vi "Calculate Channel Value.vi"(9 "Digital":bool=TRUE, 10 "Remaining Time":dbl, 11 "Step Settings":T1) -> (3 "Values to Write":dbl[](array[numeric]))   [LabVIEW 2020, in "Sequencer with Output Values.lvlib" / "Sequencer with Output Values.lvclass"]
uses:
  Sequencer with Output Values.lvclass
  Step Settings.ctl
  Global Strings.vi
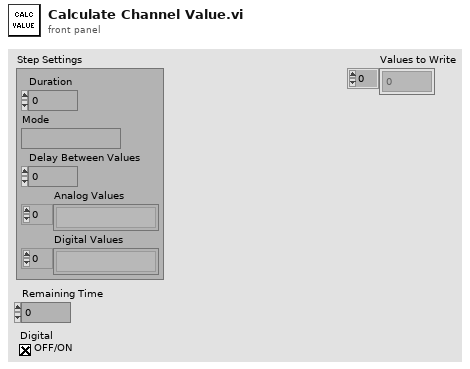
[diagram p1: front panel]
types:
  T1 = typedef "Sequencer with Output Values.lvlib/Sequencer with Output Values.lvclass/Step Settings.ctl" = cluster{"Duration":dbl, "Mode":string, "Delay Between Values":dbl, "Analog Values":string[], "Digital Values":string[]}
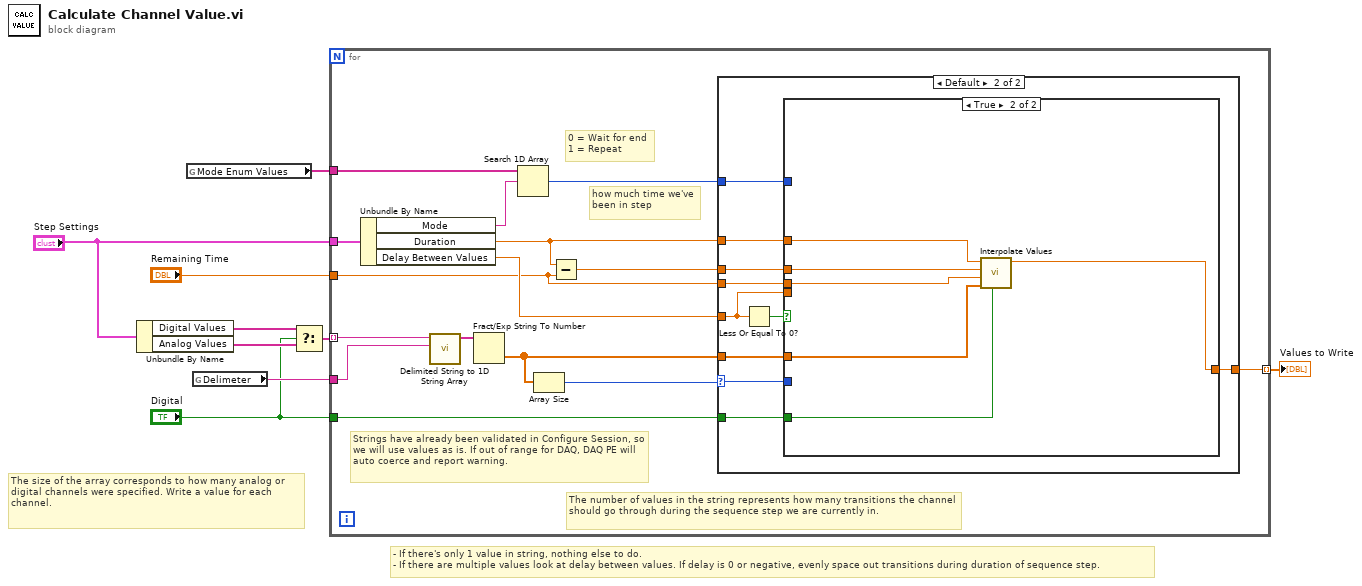
[diagram p0: block diagram]
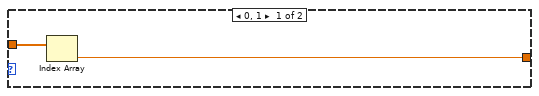
[diagram p2: hidden frame]
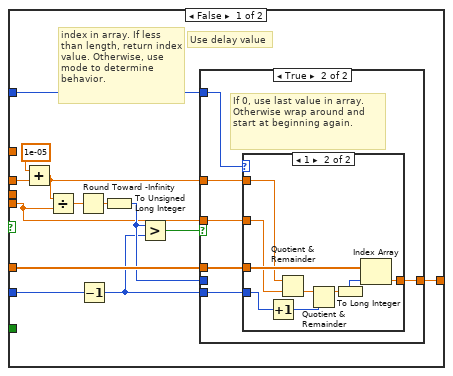
[diagram p3: hidden frame]
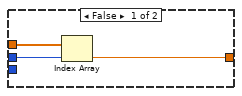
[diagram p4: hidden frame]
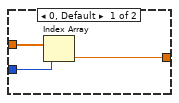
[diagram p5: hidden frame]
diagram:
  # "The size of the array corresponds to how many analog or digital channels were specified. Write a value for each channel."
  # "- If there's only 1 value in string, nothing else to do. \n- If there are multiple values look at delay between values. If delay is 0 or negative, evenly space out transitions during duration of sequence step."
  n1 = Unbundle By Name("Step Settings") -> ("Digital Values"=w5:string[], "Analog Values"=w4:string[])
  n2 = global read "Global Strings.vi" "Mode Enum Values"() -> (w7:string[])
  n3 = global read "Global Strings.vi" "Delimeter"() -> (w9:string)
  n4 = Select(t=w5, s="Digital", f=w4) -> (s? t:f=w1:string[])
  n5 = for {
    tunnel: w1 -> [w24] mode=indexing
    tunnel: w9 -> [w23]
    tunnel: "Digital" -> [w18]
    tunnel: "Step Settings" -> [w17]
    tunnel: "Remaining Time" -> [w14]
    tunnel: w7 -> [w13]
    tunnel: [w10] -> w2 mode=indexing
    # "The number of values in the string represents how many transitions the channel should go through during the sequence step we are currently in."
    # "Strings have already been validated in Configure Session, so we will use values as is. If out of range for DAQ, DAQ PE will auto coerce and report warning."
    # "how much time we've been in step"
    # "0 = Wait for end\n1 = Repeat"
    n6 = Unbundle By Name(w17) -> ("Mode"=w12:string, "Duration"=w16:dbl, "Delay Between Values"=w15:dbl)
    n7 = call <vilib>:"Delimited String to 1D String Array.vi"("delimiter"=w23, "delimited string"=w24) -> ("string array"=w22:string[])  [unwired: 9 in]
    n8 = Fract/Exp String To Number(string=w22) -> (number=w19:dbl[])  [unwired: 3 in, 1 out]
    n9 = Search 1D Array(1D array=w13, element=w12) -> (index of element=w11:i32)  [unwired: 1 in]
    n10 = Array Size(array=w19) -> (size(s)=w20:i32)
    n11 = Subtract(x=w16, y=w14) -> (x-y=w21:dbl)
    n12 = case shown="Default" w20 {
      selector: w20 -> [_ w31]
      tunnel: w19 -> [w26 w35]
      tunnel: [w25 w30] -> w10
      tunnel: w15 -> [_ w33]
      tunnel: w21 -> [_ w34]
      tunnel: w11 -> [_ w32]
      tunnel: w16 -> [_ w29]
      tunnel: w18 -> [_ w28]
      tunnel: w14 -> [_ w27]
      frame 0, 1 {
        n13 = Index Array(array=w26) -> (element=w25:dbl)  [unwired: 1 in]
      }
      frame Default {
        n14 = Less Or Equal To 0?(x=w33) -> (x <= 0?=w36:bool)
        n15 = case shown="True" w36 {
          tunnel: w35 -> [w47 w72]
          tunnel: w34 -> [w39 w74]
          tunnel: w33 -> [w41 _]
          tunnel: w32 -> [w43 _]
          tunnel: w31 -> [w49 _]
          tunnel: [w44 w76] -> w30
          tunnel: w29 -> [_ w75]
          tunnel: w28 -> [_ w71]
          tunnel: w27 -> [_ w73]
          frame False {
            # "Use delay value"
            # "index in array. If less than length, return index value. Otherwise, use mode to determine behavior."
            n16 = Add(x=1e-05, y=w39) -> (x+y=w37:dbl)
            n17 = Divide(x=w37, y=w41) -> (x/y=w40:dbl)
            n18 = Round Toward -Infinity(1:w40) -> (0:w46:dbl)
            n19 = Decrement(x=w49) -> (x-1=w42:i32)
            n20 = To Unsigned Long Integer(number=w46) -> (unsigned 32bit integer=w45:u32)
            n21 = Greater?(x=w45, y=w42) -> (0:w48:bool)
            n22 = case shown="True" w48 {
              tunnel: w47 -> [w52 w57]
              tunnel: w45 -> [w51 _]
              tunnel: [w50 w55] -> w44
              tunnel: w43 -> [_ w58]
              tunnel: w42 -> [_ w56]
              tunnel: w41 -> [_ w54]
              tunnel: w37 -> [_ w53]
              frame False {
                n23 = Index Array(array=w52, index=w51) -> (element=w50:dbl)
              }
              frame True {
                # "If 0, use last value in array. Otherwise wrap around and start at beginning again."
                n24 = case shown="1" w58 {
                  tunnel: w57 -> [w61 w70]
                  tunnel: w56 -> [w60 w67]
                  tunnel: [w59 w69] -> w55
                  tunnel: w54 -> [_ w63]
                  tunnel: w53 -> [_ w62]
                  frame 0, Default {
                    n25 = Index Array(array=w61, index=w60) -> (element=w59:dbl)
                  }
                  frame 1 {
                    n26 = Increment(x=w67) -> (x+1=w66:i32)
                    n27 = Quotient & Remainder(x=w62, y=w63) -> (floor(x/y)=w68:dbl)  [unwired: 1 out]
                    n28 = Quotient & Remainder(x=w68, y=w66) -> (x-y*floor(x/y)=w65:dbl)  [unwired: 1 out]
                    n29 = To Long Integer(number=w65) -> (32bit integer=w64:i32)
                    n30 = Index Array(array=w70, index=w64) -> (element=w69:dbl)
                  }
                }
              }
            }
          }
          frame True {
            n31 = call "Interpolate Values.vi"("Digital"=w71, "Values"=w72, "Remaining Time"=w73, "Time in Step"=w74, "Duration"=w75) -> ("Value Out"=w76:dbl)  [unwired: 6 in]
          }
        }
      }
    }
  }
  "Values to Write" <- w2
